vi "Main.vi"(9 "Sub Panel":refnum<vi>, 11 "Module Admin":refnum<class "Delacor_lib_QMH_Module Admin.lvclass">) -> ()   [LabVIEW 2020, in "Acquisition.lvlib"]
doc: "This template is based off of the Queued Message Handler design pattern and the Queued Message Handler project template that ships with LabVIEW.\n\nThe main difference is that the queue is private to this module and communication between modules is performed via Broadcast and Request events.\n\nRequest events are wrapped in public API methods and are handled in the Event Handling Loop (EHL) of this VI. Any module can register for Broadcast events sent by this module. The EHL generates messages based on user interface actions.\n\nThe Message Handling Loop (MHL) processes messages generated by the EHL, or by other messages. The messages are string values, so new messages can be added easily to the Message Cases case structure in the MHL. Each message cluster can also provide an optional value for Message Data, which is a variant that can be converted to whatever message-specific data is required.\n_____\nBased on Delacor QMH Project Template 5.0.0.82."
uses:
  Acquisition.lvlib
  <vilib>/Delacor/Delacor QMH/Libraries/Module Admin_class/Delacor_lib_QMH_Module Admin.lvclass
  Module Data--cluster.ctl
  <vilib>/userDefined/High Color/IMAQdx.ctl
  Stop Argument--cluster.ctl
  <vilib>/Delacor/Delacor QMH/Libraries/Message Queue_class/Delacor_lib_QMH_Message Queue.lvclass/Delacor_lib_QMH_Message Queue.ctl
  <vilib>/Delacor/Delacor QMH/Libraries/Module Admin_class/Delacor_lib_QMH_Module Admin.lvclass/Delacor_lib_QMH_Module Admin.ctl
  Start Acquisition Argument--cluster.ctl
  Stop Acquisition Argument--cluster.ctl
  <vilib>/Delacor/Delacor QMH/Libraries/Message Queue_class/Delacor_lib_QMH_Enqueue Message (Single).vi
  <vilib>/Delacor/Delacor QMH/Libraries/Module Admin_class/Delacor_lib_QMH_Get External Launch.vi
  <vilib>/Utility/error.llb/Error Cluster From Error Code.vi
  <vilib>/ErrorRing/Error Ring.xnode
  <vilib>/Delacor/Delacor QMH/Libraries/Message Queue_class/Delacor_lib_QMH_Message Queue.lvclass
  <vilib>/vision/driver/NI_Vision_Acquisition_Software.lvlib
  Analisis/Analisis.lvlib
panel:
  out "Image":T1(plugin-control)
  out "error out":errorcluster
  out "Status":string
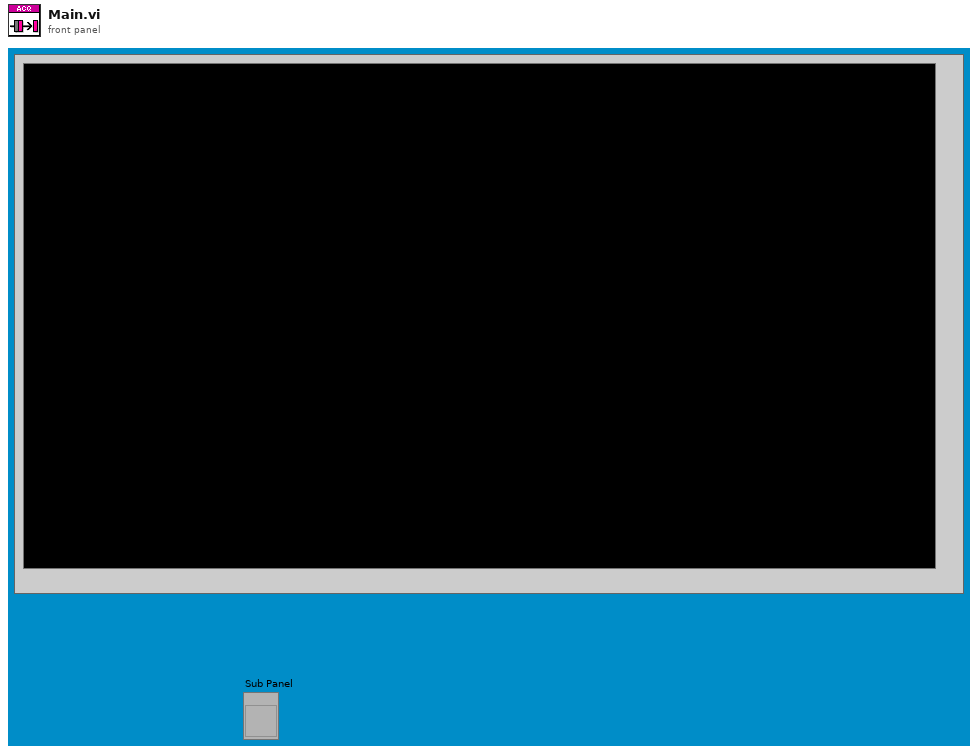
[diagram p1: front panel]
types:
  T1 = typedef "IMAQ Image.ctl" = refnum<image>
  T2 = typedef "Acquisition.lvlib/Request Events--cluster.ctl" = cluster{"Stop Module":refnum<user-event>, "Show Panel":refnum<user-event>, "Hide Panel":refnum<user-event>, "Get Module Execution Status":refnum<user-event>, "Show Diagram":refnum<user-event>, "Start Acquisition":refnum<user-event>, "Stop Acquisition":refnum<user-event>}
  T3 = typedef "IMAQdx.ctl" = refnum<k21>
  T4 = typedef "Acquisition.lvlib/Module Data--cluster.ctl" = cluster{"Status":string}
  T5 = typedef "Acquisition.lvlib/Start Acquisition Argument--cluster.ctl" = cluster{"Boolean":bool}
  T6 = typedef "Acquisition.lvlib/Stop Acquisition Argument--cluster.ctl" = cluster{"Boolean":bool}
  T7 = enum32{"invalid lock state", "Not Locked", "Locked (No Password)", "Password-protected"}
  T8 = typedef "Acquisition.lvlib/Stop Argument--cluster.ctl" = cluster{"Origin":string, "Exit via Stop Module Req?":bool, "Wait for Module to stop?":bool}
  T9 = enum32{"Invalid", "Standard", "Closed", "Hidden", "Minimized", "Maximized"}
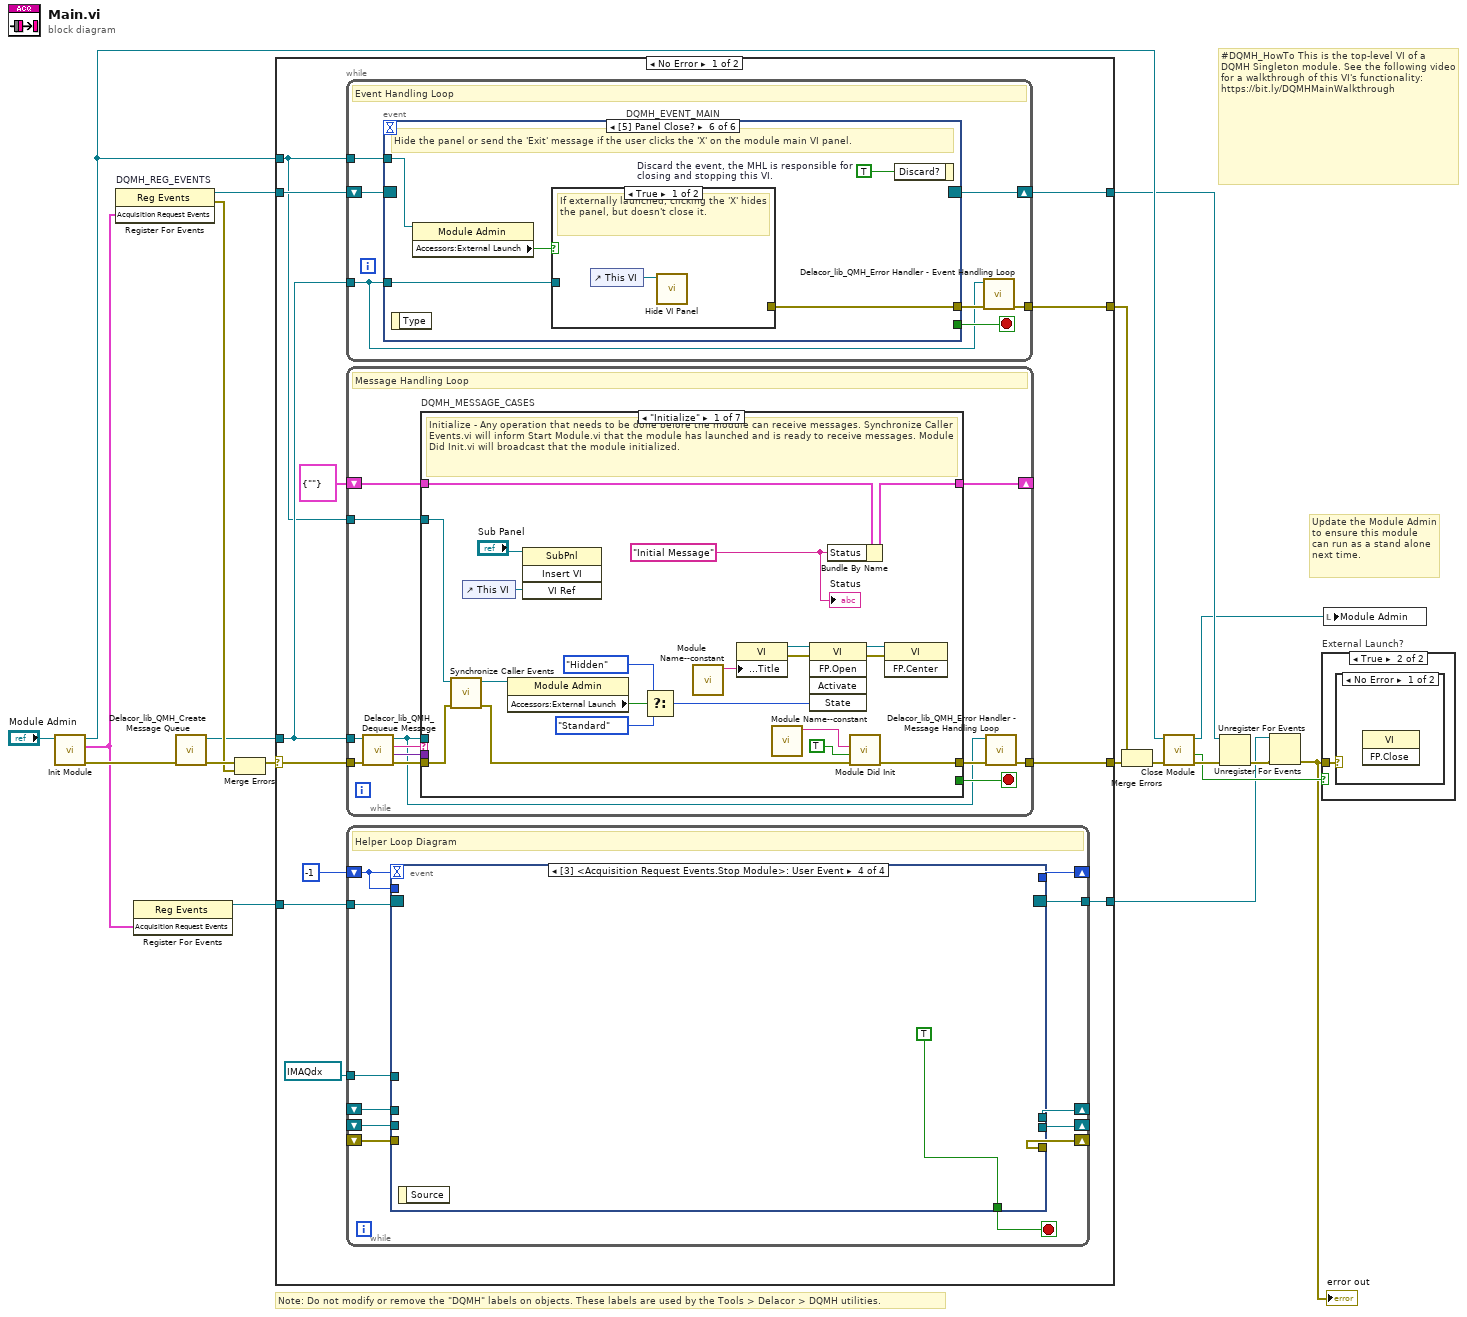
[diagram p0: block diagram]
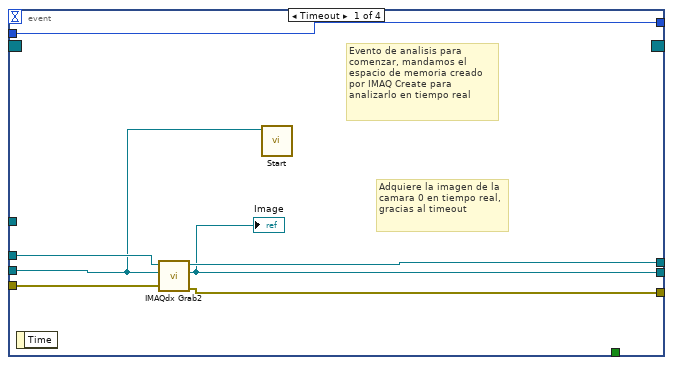
[diagram p2: hidden frame]
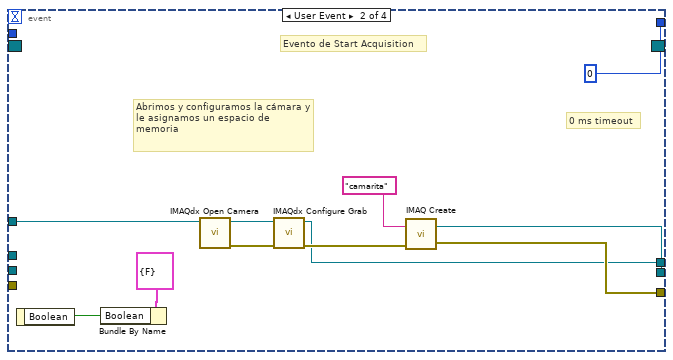
[diagram p3: hidden frame]
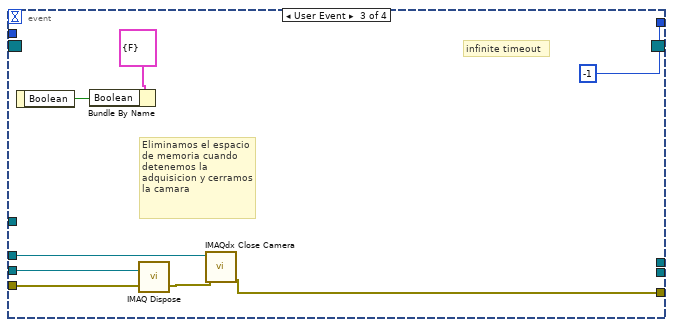
[diagram p4: hidden frame]
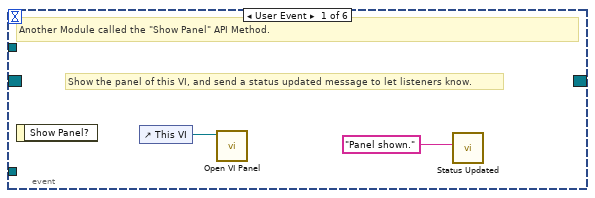
[diagram p5: hidden frame]
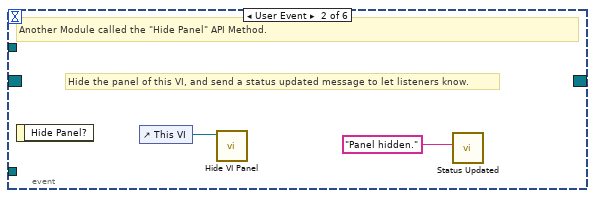
[diagram p6: hidden frame]
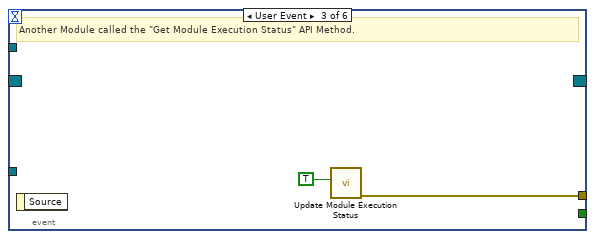
[diagram p7: hidden frame]
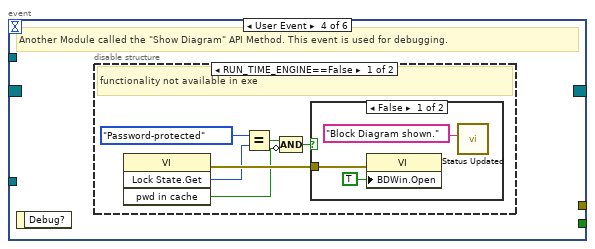
[diagram p8: hidden frame]
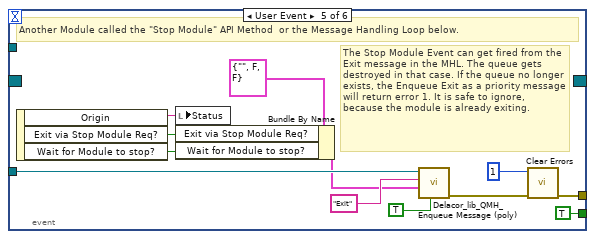
[diagram p11: hidden frame]
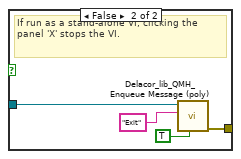
[diagram p12: hidden frame]
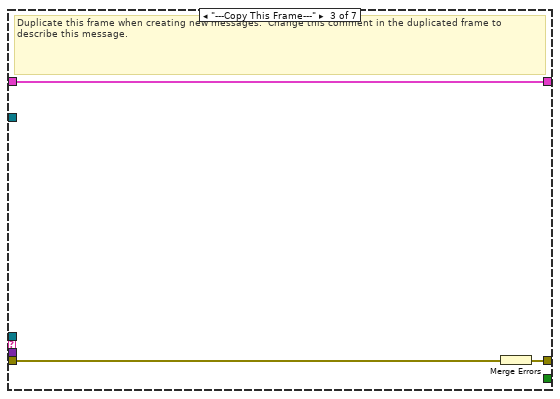
[diagram p14: hidden frame]
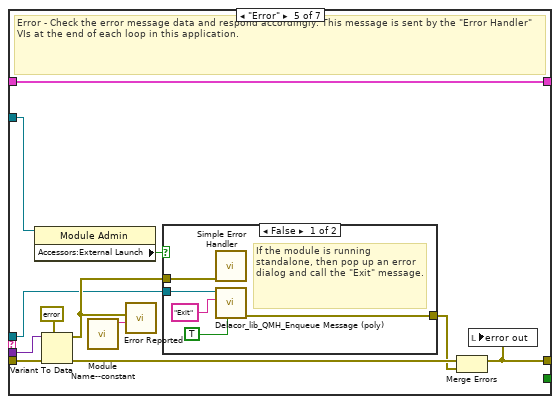
[diagram p16: hidden frame]
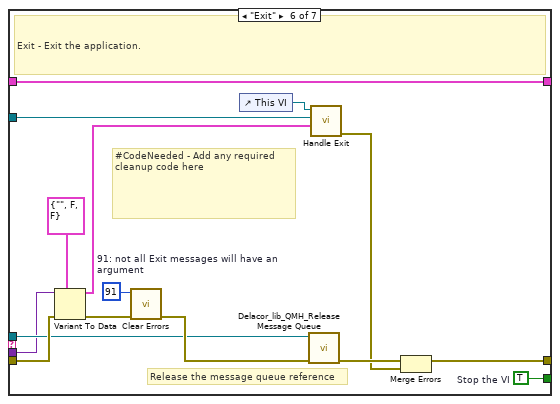
[diagram p18: hidden frame]
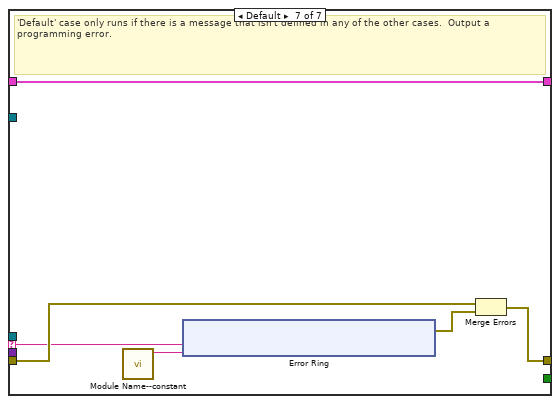
[diagram p19: hidden frame]
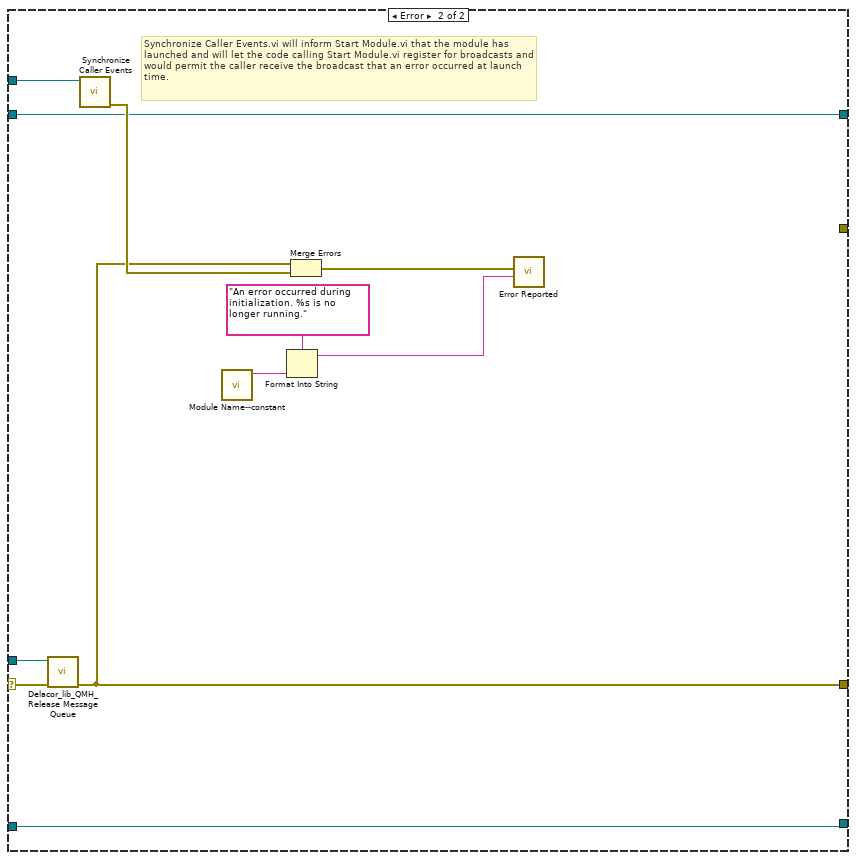
[diagram p20: hidden frame]
diagram:
  # "#DQMH_HowTo This is the top-level VI of a DQMH Singleton module. See the following video for a walkthrough of this VI's functionality: https://bit.ly/DQMHMainWalkthrough"
  # "Note: Do not modify or remove the \"DQMH\" labels on objects. These labels are used by the Tools > Delacor > DQMH utilities."
  # "Update the Module Admin to ensure this module can run as a stand alone next time."
  n1 = call "Init Module.vi"("Singleton Module Admin in"="Module Admin") -> ("error out"=w19:errorcluster, "Acquisition Request Events"=w5:T2, "Singleton Module Admin out"=w12:refnum<class "Delacor_lib_QMH_Module Admin.lvclass">)  [unwired: 8 in]
  n2 = register-events "DQMH_REG_EVENTS"(w5) -> (reference out=w10:refnum<event-registration>, error out=w13:errorcluster)  [unwired: 2 in]
  n3 = register-events(w5) -> (reference out=w2:refnum<event-registration>)  [unwired: 2 in, 1 out]
  n4 = call <vilib>:"Delacor_lib_QMH_Create Message Queue.vi"("error in (no error)"=w19) -> ("error out"=w15:errorcluster, "Message Queue"=w9:refnum<class "Delacor_lib_QMH_Message Queue.lvclass">)  [unwired: 9 in]
  n5 = Merge Errors(w15, w13) -> (w14:errorcluster)
  n6 = case shown="No Error" w14 {
    selector: w14 -> [w30 w205]
    tunnel: [w32 w204] -> w20
    tunnel: [w29 w210] -> w11
    tunnel: w10 -> [w27 w210]
    tunnel: w9 -> [w26 w203]
    tunnel: [w31 _] -> w17
    tunnel: w12 -> [w25 w206]
    tunnel: w2 -> [w24 w202]
    tunnel: [w23 w202] -> w1
    frame No Error {
      n7 = while {
        tunnel: w26 -> [w72]
        shift-right: [w75] -> w29
        shift-left: w27 -> [w76]
        tunnel: [w77] -> w31
        tunnel: w25 -> [w73]
        stop <- w74 stop-if-true
        # "Event Handling Loop"
        n8 = event "DQMH_EVENT_MAIN" shown="[5] Panel Close?" {
          selector: w76 -> [_ _ _ _ _ _]
          dyn-events: [_ _ _ _ _ _] -> w75
          timeout: _ -> [_ _ _ _ _ _]
          tunnel: [_ _ _ _ TRUE ("Discard?") _] -> w74
          tunnel: w72 -> [_ _ _ _ w101 w108]
          tunnel: [_ _ w84 _ w104 w110] -> w78
          tunnel: w73 -> [_ _ _ _ _ w107]
          event User Event {
            # "Show the panel of this VI, and send a status updated message to let listeners know."
            # "Another Module called the \"Show Panel\" API Method."
            n9 = event-data() -> ()  [unwired: 1 in, 1 out]
            n10 = control-ref of="This VI"() -> (w80:refnum<vi>)
            n11 = call "Open VI Panel.vi"("VI"=w80) -> ()  [unwired: 10 in, 1 out]
            n12 = call "Status Updated.vi"("Status"="Panel shown." ("format string")) -> ()  [unwired: 10 in, 1 out]
          }
          event User Event {
            # "Hide the panel of this VI, and send a status updated message to let listeners know."
            # "Another Module called the \"Hide Panel\" API Method."
            n13 = event-data() -> ()  [unwired: 1 in, 1 out]
            n14 = control-ref of="This VI"() -> (w82:refnum<vi>)
            n15 = call "Hide VI Panel.vi"("VI"=w82) -> ()  [unwired: 10 in, 1 out]
            n16 = call "Status Updated.vi"("Status"="Panel hidden." ("format string")) -> ()  [unwired: 10 in, 1 out]
          }
          event User Event {
            # "Another Module called the \"Get Module Execution Status\" API Method."
            n17 = event-data() -> ()  [unwired: 1 in, 1 out]
            n18 = call "Update Module Execution Status.vi"("Running?"=TRUE) -> ("error out"=w84:errorcluster)  [unwired: 10 in]
          }
          event User Event {
            # "Another Module called the \"Show Diagram\" API Method. This event is used for debugging."
            n19 = event-data() -> ()  [unwired: 1 in, 1 out]
            n20 = disable-structure shown="RUN_TIME_ENGINE==False" {
              frame condition #0 (active) {
                # "functionality not available in exe"
                n21 = invoke class="VI" method="Lock State.Get"() -> (error out=w90:errorcluster, "Get Lock State"=w89:T7, "pwd in cache"=w86:bool)  [unwired: 4 in, 1 out]
                n22 = Equal?(x=T7."Password-protected", y=w89) -> (x = y?=w87:bool)
                n23 = Compound Arithmetic op=AND(w87, invert w86) -> (w85:bool)
                n24 = case shown="False" w85 {
                  tunnel: w90 -> [w93 _]
                  frame False {
                    n25 = property class="VI"(error in=w93, "BDWin.Open"=TRUE ("Block Diagram Window:Open")) -> ()  [unwired: 1 in, 2 out]
                    n26 = call "Status Updated.vi"("Status"="Block Diagram shown." ("format string")) -> ()  [unwired: 10 in, 1 out]
                  }
                  frame True {
                    # "Password-protected VI, and the password is not in the cache. Do not show the diagram."
                  }
                }
              }
              frame condition #1 {
              }
            }
          }
          event User Event {
            # "The Stop Module Event can get fired from the Exit message in the MHL. The queue gets destroyed in that case. If the queue no longer exists, the Enqueue Exit as a priority message will return error 1. It is safe to ignore, because the module is already exiting."
            # "Another Module called the \"Stop Module\" API Method  or the Message Handling Loop below."
            n27 = event-data() -> ("Origin"=w100:string, "Exit via Stop Module Req?"=w96:bool, "Wait for Module to stop?"=w95:bool)  [unwired: 1 in]
            n28 = local write "Status"(w100) -> ()
            n29 = Bundle By Name(cluster=T8 {"Origin"="", "Exit via Stop Module Req?"=FALSE, "Wait for Module to stop?"=FALSE} ("Stop Argument"), "Exit via Stop Module Req?"=w96, "Wait for Module to stop?"=w95) -> (w94:T8)
            n30 = call-poly <vilib>:"Delacor_lib_QMH_Enqueue Message (poly).vi"("Priority Message? (F)"=TRUE, "Message Data"=w94, "Message"="Exit", "Message Queue in"=w101) -> ("error out"=w105:errorcluster)  [unwired: 6 in, 1 out]
            n31 = call <vilib>:"Clear Errors.vi"("error in (no error)"=w105, "specific error code to clear (0: all)"=1) -> ("error out"=w104:errorcluster)  [unwired: 4 in, 1 out]
          }
          event Panel Close? {
            w109 = TRUE  # Discard the event, the MHL is responsible for closing and stopping this VI.
            # "Hide the panel or send the 'Exit' message if the user clicks the 'X' on the module main VI panel."
            n32 = event-data() -> ()  [unwired: 1 in, 1 out]
            n33 = property class="Module Admin"(reference=w107) -> ("Accessors:External Launch"=w106:bool)  [unwired: 1 in, 2 out]
            n34 = case shown="True" w106 {
              tunnel: w108 -> [_ w114]
              tunnel: [_ w115] -> w110
              frame True {
                # "If externally launched, clicking the 'X' hides the panel, but doesn't close it."
                n35 = control-ref of="This VI"() -> (w111:refnum<vi>)
                n36 = call "Hide VI Panel.vi"("VI"=w111) -> ()  [unwired: 10 in, 1 out]
              }
              frame False {
                # "If run as a stand-alone VI, clicking the panel 'X' stops the VI."
                n37 = call-poly <vilib>:"Delacor_lib_QMH_Enqueue Message (poly).vi"("Priority Message? (F)"=TRUE, "Message"="Exit", "Message Queue in"=w114) -> ("error out"=w115:errorcluster)  [unwired: 7 in, 1 out]
              }
            }
            n38 = event-data("Discard?"=w109) -> ()  [unwired: 1 in, 1 out]
          }
        }
        n39 = call-dynamic "Delacor_lib_QMH_Error Handler - Event Handling Loop.vi"("error in (no error)"=w78, "Message Queue in"=w72) -> ("dup error in"=w77:errorcluster)  [unwired: 8 in, 1 out]
      }
      n40 = while {
        tunnel: w26 -> [w118]
        shift-right: [w122] -> _
        shift-left: T4 {"Status"=""} ("Data Cluster") -> [w123]
        tunnel: w30 -> [w126]
        tunnel: [w124] -> w32
        tunnel: w25 -> [w116]
        stop <- w121 stop-if-true
        # "Message Handling Loop"
        n41 = call-dynamic "Delacor_lib_QMH_Dequeue Message.vi"("error in (no error)"=w126, "Message Queue in"=w118) -> ("error out"=w125:errorcluster, "Message Data"=w119:variant, "Message"=w120:string, "Message Queue out"=w117:refnum<class "Delacor_lib_QMH_Message Queue.lvclass">)  [unwired: 6 in]
        n42 = case "DQMH_MESSAGE_CASES" shown="\"Initialize\"" w120 {
          selector: w120 -> [_ _ _ _ _ _ w189]
          tunnel: w117 -> [_ _ _ _ w159 w181 _]
          tunnel: w125 -> [w146 w150 w153 w155 w166 w187 w191]
          tunnel: [w144 w150 w152 w155 w162 w184 w192] -> w127
          tunnel: w123 -> [w135 w149 w151 w154 w161 w180 w190]
          tunnel: [w134 w149 w151 w154 w161 w180 w190] -> w122
          tunnel: [_ _ _ _ _ w179 _] -> w121
          tunnel: w119 -> [_ _ _ _ w160 w178 _]
          tunnel: w116 -> [w136 _ _ _ w158 w173 _]
          frame "Initialize" {
            w130 = "Initial Message" ("Initial Message")
            # "Initialize - Any operation that needs to be done before the module can receive messages. Synchronize Caller Events.vi will inform Start Module.vi that the module has launched and is ready to receive messages. Module Did Init.vi will broadcast that the module initialized."
            n43 = call "Synchronize Caller Events.vi"("error in (no error)"=w146, "Singleton Module Admin in"=w136) -> ("error out"=w145:errorcluster, "Singleton Module Admin out"=w131:refnum<class "Delacor_lib_QMH_Module Admin.lvclass">)  [unwired: 8 in]
            n44 = control-ref of="This VI"() -> (w128:refnum<vi>)
            n45 = property class="Module Admin"(reference=w131) -> ("Accessors:External Launch"=w140:bool)  [unwired: 1 in, 2 out]
            n46 = invoke class="SubPnl" method="Insert VI"(reference="Sub Panel", "VI Ref"=w128) -> ()  [unwired: 2 in, 4 out]
            n47 = Select(t=T9."Hidden" ("State"), s=w140, f=T9."Standard" ("State")) -> (s? t:f=w137:T9)
            n48 = call "Module Name--constant.vi"() -> ("Module Name"=w143:string)  [unwired: 11 in]
            n49 = property class="VI"("Front Panel.Title"=w143) -> (reference out=w142:refnum<vi>, error out=w148:errorcluster)  [unwired: 2 in]
            n50 = call "Module Name--constant.vi"() -> ("Module Name"=w132:string)  [unwired: 11 in]
            n51 = invoke class="VI" method="FP.Open"(reference=w142, error in=w148, "State"=w137) -> (reference out=w141:refnum<vi>, error out=w147:errorcluster)  [unwired: 2 in, 3 out]
            n52 = Bundle By Name(cluster=w135, "Status"=w130) -> (w134:T4)
            n53 = call "Module Did Init.vi"("error in (no error)"=w145, "Initialized?"=TRUE, "Origin"=w132) -> ("error out"=w144:errorcluster)  [unwired: 8 in]
            n54 = invoke class="VI" method="FP.Center"(reference=w141, error in=w147) -> ()  [unwired: 1 in, 3 out]
            "Status" <- w130
          }
          frame "--- Module Specific ---" {
            # "Separator -- The following cases handle messages specific to this Module."
          }
          frame "---Copy This Frame---" {
            # "Duplicate this frame when creating new messages.  Change this comment in the duplicated frame to describe this message."
            n55 = Merge Errors(w153) -> (w152:errorcluster)
          }
          frame "--- Exit and Error Handling---" {
            # "Separator - The following cases handle errors and exit messages."
          }
          frame "Error" {
            # "Error - Check the error message data and respond accordingly. This message is sent by the \"Error Handler\" VIs at the end of each loop in this application."
            n56 = property class="Module Admin"(reference=w158) -> ("Accessors:External Launch"=w157:bool)  [unwired: 1 in, 2 out]
            n57 = Variant To Data(error in=w166, type=errorcluster {"status"=FALSE, "code"=0, "source"=""} ("error constant"), Variant=w160) -> (data=w167:errorcluster, error out=w164:errorcluster)
            n58 = call "Module Name--constant.vi"() -> ("Module Name"=w156:string)  [unwired: 11 in]
            n59 = call "Error Reported.vi"("Additional Information"=w156, "Error"=w167) -> ()  [unwired: 9 in, 1 out]
            n60 = case shown="False" w157 {
              tunnel: [w172 _] -> w163
              tunnel: w159 -> [w170 _]
              tunnel: w167 -> [w171 _]
              frame False {
                # "If the module is running standalone, then pop up an error dialog and call the \"Exit\" message."
                n61 = call <vilib>:"Simple Error Handler.vi"("error in (no error)"=w171) -> ()  [unwired: 4 in, 5 out]
                n62 = call-poly <vilib>:"Delacor_lib_QMH_Enqueue Message (poly).vi"("Priority Message? (F)"=TRUE, "Message"="Exit", "Message Queue in"=w170) -> ("error out"=w172:errorcluster)  [unwired: 7 in, 1 out]
              }
              frame True {
                # "If the module was launched externally, calling the Error Reported broadcast VI is the only action performed by the \"Error\" message. The module's caller can then process the error appropriately."
              }
            }
            n63 = Merge Errors(w164, w163) -> (w162:errorcluster)
            n64 = local write "error out"(w162) -> ()
          }
          frame "Exit" {
            w177 = 91  # 91: not all Exit messages will have an argument
            w179 = TRUE  # Stop the VI
            # "Release the message queue reference"
            # "#CodeNeeded - Add any required cleanup code here"
            # "Exit - Exit the application."
            n65 = Variant To Data(error in=w187, type=T8 {"Origin"="", "Exit via Stop Module Req?"=FALSE, "Wait for Module to stop?"=FALSE} ("Stop Argument"), Variant=w178) -> (data=w175:T8, error out=w183:errorcluster)
            n66 = call <vilib>:"Clear Errors.vi"("error in (no error)"=w183, "specific error code to clear (0: all)"=w177) -> ("error out"=w186:errorcluster)  [unwired: 4 in, 1 out]
            n67 = control-ref of="This VI"() -> (w174:refnum<vi>)
            n68 = call-dynamic "Delacor_lib_QMH_Release Message Queue.vi"("error in (no error)"=w186, "Message Queue"=w181) -> ("error out"=w185:errorcluster)  [unwired: 9 in]
            n69 = call "Handle Exit.vi"("Stop Argument"=w175, "Admin in"=w173, "VI reference"=w174) -> ("error out"=w182:errorcluster)  [unwired: 7 in, 1 out]
            n70 = Merge Errors(w185, w182) -> (w184:errorcluster)
          }
          frame Default {
            # "'Default' case only runs if there is a message that isn't defined in any of the other cases.  Output a programming error."
            n71 = call "Module Name--constant.vi"() -> ("Module Name"=w188:string)  [unwired: 11 in]
            n72 = xnode "Error Ring"("parameter 0"=w189, "parameter 1"=w188) -> ("error out"=w193:errorcluster)
            n73 = Merge Errors(w191, w193) -> (w192:errorcluster)
          }
        }
        n74 = call-dynamic "Delacor_lib_QMH_Error Handler - Message Handling Loop.vi"("error in (no error)"=w127, "Message Queue in"=w117) -> ("dup error in"=w124:errorcluster)  [unwired: 8 in, 1 out]
      }
      n75 = while {
        tunnel: w24 -> [w44]
        tunnel: [w43] -> w23
        shift-right: [w41] -> _
        shift-left: -1 -> [w42]
        tunnel: T3 "cam0" ("Session In") -> [w40]
        shift-right: [w39] -> _
        shift-left: _ -> [w37]
        shift-right: [w36] -> _
        shift-left: _ -> [w35]
        shift-right: [w34] -> _
        shift-left: _ -> [w33]
        stop <- w38 stop-if-true
        # "Helper Loop Diagram"
        n76 = event shown="[3] <Acquisition Request Events.Stop Module>: User Event" {
          selector: w44 -> [_ _ _ _]
          dyn-events: [_ _ _ _] -> w43
          timeout: w42 -> [_ _ _ _]
          tunnel: w42 -> [w47 _ _ _]
          tunnel: [w47 0 -1 _] -> w41
          tunnel: w40 -> [_ w61 _ _]
          tunnel: [w48 w56 w67 _] -> w39
          tunnel: [_ _ _ TRUE] -> w38
          tunnel: w37 -> [w49 _ w69 _]
          tunnel: [w51 w54 _ _] -> w36
          tunnel: w35 -> [w50 _ w66 _]
          tunnel: [w46 w52 _ _] -> w34
          tunnel: w33 -> [w45 _ w63 _]
          event Timeout {
            # "Evento de analisis para comenzar, mandamos el espacio de memoria creado por IMAQ Create para analizarlo en tiempo real"
            # "Adquiere la imagen de la camara 0 en tiempo real, gracias al timeout"
            n77 = event-data() -> ()  [unwired: 1 in, 1 out]
            n78 = call <vilib>:"IMAQdx Grab2.vi"("error in"=w49, "Image In"=w45, "Session In"=w50) -> ("error out"=w48:errorcluster, "Image Out"=w46:T1, "Session Out"=w51:T3)  [unwired: 5 in, 1 out]
            "Image" <- w46
            n79 = call "Start.vi"("Image In"=w45) -> ()  [unwired: 10 in, 1 out]
          }
          event User Event {
            # "Evento de Start Acquisition"
            # "Abrimos y configuramos la cámara y le asignamos un espacio de memoria"
            # "0 ms timeout"
            n80 = event-data() -> ("Boolean"=w53:bool)  [unwired: 1 in]
            n81 = Bundle By Name(cluster=T5 {"Boolean"=FALSE} ("Start Acquisition Argument"), "Boolean"=w53) -> ()  [unwired: 1 out]
            n82 = call <vilib>:"IMAQdx Open Camera.vi"("Session In"=w61) -> ("error out"=w57:errorcluster, "Session Out"=w60:T3)  [unwired: 9 in]
            n83 = call <vilib>:"IMAQdx Configure Grab.vi"("error in"=w57, "Session In"=w60) -> ("error out"=w58:errorcluster, "Session Out"=w54:T3)  [unwired: 8 in]
            n84 = call "IMAQ Create"("Image Name"="camarita", "error in (no error)"=w58) -> ("New Image"=w52:T1, "error out"=w56:errorcluster)  [unwired: 3 in]
          }
          event User Event {
            # "Eliminamos el espacio de memoria cuando detenemos la adquisicion y cerramos la camara"
            # "infinite timeout"
            n85 = event-data() -> ("Boolean"=w64:bool)  [unwired: 1 in]
            n86 = Bundle By Name(cluster=T6 {"Boolean"=FALSE} ("Stop Acquisition Argument"), "Boolean"=w64) -> ()  [unwired: 1 out]
            n87 = call "IMAQ Dispose"("Image"=w63, "error in (no error)"=w69) -> ("error out"=w68:errorcluster)  [unwired: 4 in]
            n88 = call <vilib>:"IMAQdx Close Camera.vi"("error in"=w68, "Session In"=w66) -> ("error out"=w67:errorcluster)  [unwired: 9 in]
          }
          event User Event {
            n89 = event-data() -> ()  [unwired: 1 in, 1 out]
          }
        }
      }
    }
    frame Error {
      # "Synchronize Caller Events.vi will inform Start Module.vi that the module has launched and will let the code calling Start Module.vi register for broadcasts and would permit the caller receive the broadcast that an error occurred at launch time."
      n90 = call-dynamic "Delacor_lib_QMH_Release Message Queue.vi"("error in (no error)"=w205, "Message Queue"=w203) -> ("error out"=w204:errorcluster)  [unwired: 9 in]
      n91 = call "Synchronize Caller Events.vi"("Singleton Module Admin in"=w206) -> ("error out"=w211:errorcluster)  [unwired: 9 in, 1 out]
      n92 = call "Module Name--constant.vi"() -> ("Module Name"=w209:string)  [unwired: 11 in]
      n93 = Format Into String(format string="An error occurred during initialization. %s is no longer running.", w209) -> (resulting string=w207:string)  [unwired: 2 in, 1 out]
      n94 = Merge Errors(w204, w211) -> (w212:errorcluster)
      n95 = call "Error Reported.vi"("Additional Information"=w207, "Error"=w212) -> ()  [unwired: 9 in, 1 out]
    }
  }
  n96 = Merge Errors(w17, w20) -> (w16:errorcluster)
  n97 = call "Close Module.vi"("error in (no error)"=w16, "Module Admin in"=w12) -> ("error out"=w18:errorcluster, "External Launch"=w6:bool, "Module Admin out"=w7:refnum<class "Delacor_lib_QMH_Module Admin.lvclass">)  [unwired: 7 in]
  n98 = Unregister For Events(event registration refnum=w11, error in=w18) -> (error out=w4:errorcluster)
  n99 = Unregister For Events(event registration refnum=w1, error in=w4) -> (error out=w3:errorcluster)
  "error out" <- w3
  n100 = case "External Launch?" shown="True" w6 {
    tunnel: w3 -> [_ w213]
    frame False {
    }
    frame True {
      n101 = case shown="No Error" w213 {
        frame No Error {
          n102 = invoke class="VI" method="FP.Close"() -> ()  [unwired: 3 in, 3 out]
        }
        frame Error {
          n103 = invoke class="VI" method="FP.Open"("Activate"=TRUE ("Activate?")) -> ()  [unwired: 4 in, 5 out]
        }
      }
    }
  }
  n104 = local write "Module Admin"(w7) -> ()
